vi "ISEG_HVBoardGUI.panel.vi"(0 "object ref":refnum<vi>, 5 "error in (no error)":errorcluster) -> (19 "error out":errorcluster)   [LabVIEW 2014, in "ISEG_HVBoardGUI.lvlib"]
doc: "This is just an example for a ISEG HV Board GUI .\n\nLicense Agreement for this software:\n\nCopyright (C)\nGesellschaft für Schwerionenforschung, GSI\nPlanckstr. 1\n64291 Darmstadt\nGermany\n\nContact: D.Beck@gsi.de \n\nThis program is free software; you can redistribute it and/or modify it under the terms of the GNU General Public License as published by the Free Software Foundation; either version 2 of the license, or (at your option) any later version.\n\nThis program is distributed in the hope that it will be useful, but WITHOUT ANYW ARRANTY; without even the implied warranty of MERCHANTABILITY or FITNESS FOR A PARTICULAR PURPOSE. See the GNU General License for more details (http://www.gnu.org).\n\nGesellschaft für Schwerionenforschung, GSI\nPlanckstr. 1, 64291 Darmstadt, Germany\nFor all questions and ideas contact: M.Richter@gsi.de, H.Brand@gsi.de or D.Beck@gsi.de.\nLast update: 18-DEC-2002"
uses:
  ISEG_HVBoardGUI.lvlib
  CSlibraries-extern/DimLVEvent/DimIndicators/DimIndicators.numericType.ctl
  CSlibraries-extern/DimLVEvent/DimIndicators/DimIndicators.anyType.ctl
  CSCore/CSSystem/CoreDefs/CoreDefs.call_type.ctl
  CSCore/BaseProcess/BaseProcess.descriptor string definition.ctl
  CSCore/CSSystem/CoreDefs/CoreDefs.rawDataType.ctl
  CSCore/CSSystem/CoreLib/CoreLib.double 2 byte array.vi
  CSCore/CSSystem/CoreLib/CoreLib.short 2 byte array.vi
  CSCore/CSSystem/CoreLib/CoreLib.string 2 byte array.vi
  CSlibraries-extern/DimLVEvent/DimIndicators/DimIndicators.lvlib
  CSCore/CSSystem/CSSystemLib/CSSystemLib.lvlib
  CSCore/CSSystem/CoreLib/CoreLib.lvlib
  CSCore/BaseProcess/BaseProcess.lvlib
  CSlibraries/UtilityLib/UtilityLib.lvlib
panel:
  out "Status":bool
  in  "Refresh":T1
  out "Refrech":bool caption="CANBUS_BUSY"
  out "On/Off_Status":bool
  in  "Event_Status":T1
  in  "SetVAll":T1
  in  "On":T1
  in  "Clear":T1
  in  "Kill":T1
  in  "RampRate":T1
  out "Device Class":dbl
  in  "DeviceClass":T1
  in  "AlarmStatus":T1
  in  "Alarm":T1
  in  "Clear":bool
  in  "SetRampRate":dbl
  in  "On":bool
  out "Alarm":bool
  out "AlarmStatus":u16 caption="Alarming" format="%.0b"
  in  "SetV All channels":dbl
  in  "call cluster in":T2={"Object"="", "Selector"="", "CallType"=enum."synchronous", "Async Object"="", "Async Selector"="", "Data Descriptor"="", "Data"=[], "Error #"=0, "Expire"=0}
  in  "KillStatus":T1
  in  "Kill":bool
  out "Status":bool
  in  "BoardTemp":T1
  in  "HardwareVLimit":T1
  in  "Status":T1
  in  "NrOfCh":T1
  in  "DeviceID":T5
  out "loop counter":i32
  in  "DeviceState":T1
  out "Object Name":string
  out "Board":i16
  out "System Name":string
  out "Temp":dbl
  out "NrOfCh":u16
  out "HVMax":dbl format="%#_f"
  out "BdStatus":u16 caption="Status" format="%016b"
  out "DeviceID":string
  out "time stamp":timestamp
  in  "stop":bool
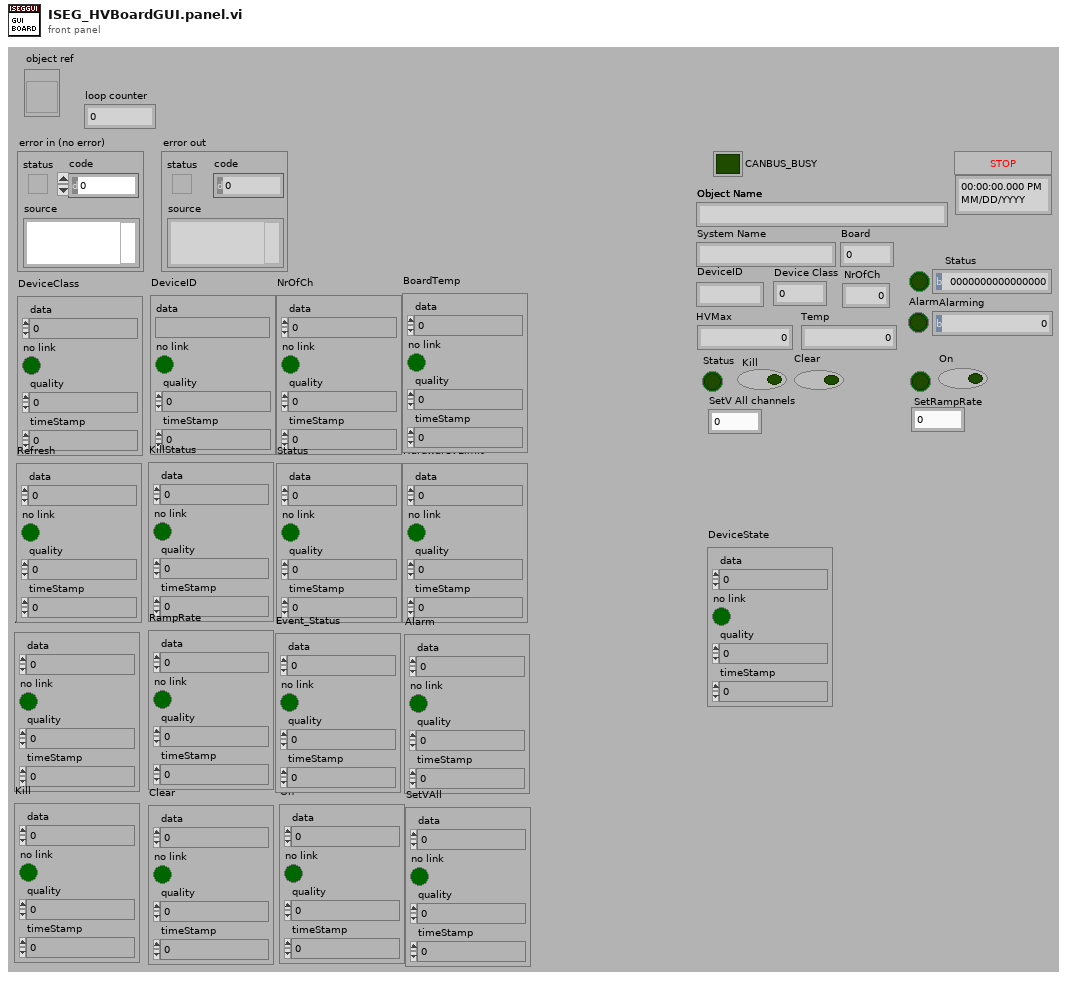
[diagram p1: front panel]
types:
  T1 = typedef "DimIndicators.lvlib/DimIndicators.numericType.ctl" = cluster{"data":dbl, "no link":bool, "quality":i32, "timeStamp":dbl}
  T2 = typedef "CoreDefs.call_type.ctl" = cluster{"Object":string, "Selector":string, "CallType":enum16{"simple", "synchronous", "asynchronous"}, "Async Object":string, "Async Selector":string, "Data Descriptor":T3, "Data":T4, "Error #":i32, "Expire":u32}
  T3 = typedef "BaseProcess.lvlib/BaseProcess.descriptor string definition.ctl" = string
  T4 = typedef "CoreDefs.rawDataType.ctl" = i8[]
  T5 = typedef "DimIndicators.lvlib/DimIndicators.anyType.ctl" = cluster{"data":string, "no link":bool, "quality":i32, "timeStamp":dbl}
  T6 = typedef "ISEG_HVBoardGUI.lvlib/ISEG_HVBoardGUI.i attribute.ctl" = cluster{"System Name":string, "Slot":i16, "Object Name":string, "Prefix":string}
  T7 = typedef "DeviceBase.lvlib/DeviceBase.deviceState.ctl" = i16
  T8 = typedef "UtilityLib.lvlib/UtilityLib.valueStatus.ctl" = enum16{"no info available", "stand by/off", "on", "warning", "alarm/malfunction", "not implemented", "user action required", "important information", "system default", "control default", "indicator default", "button default"}
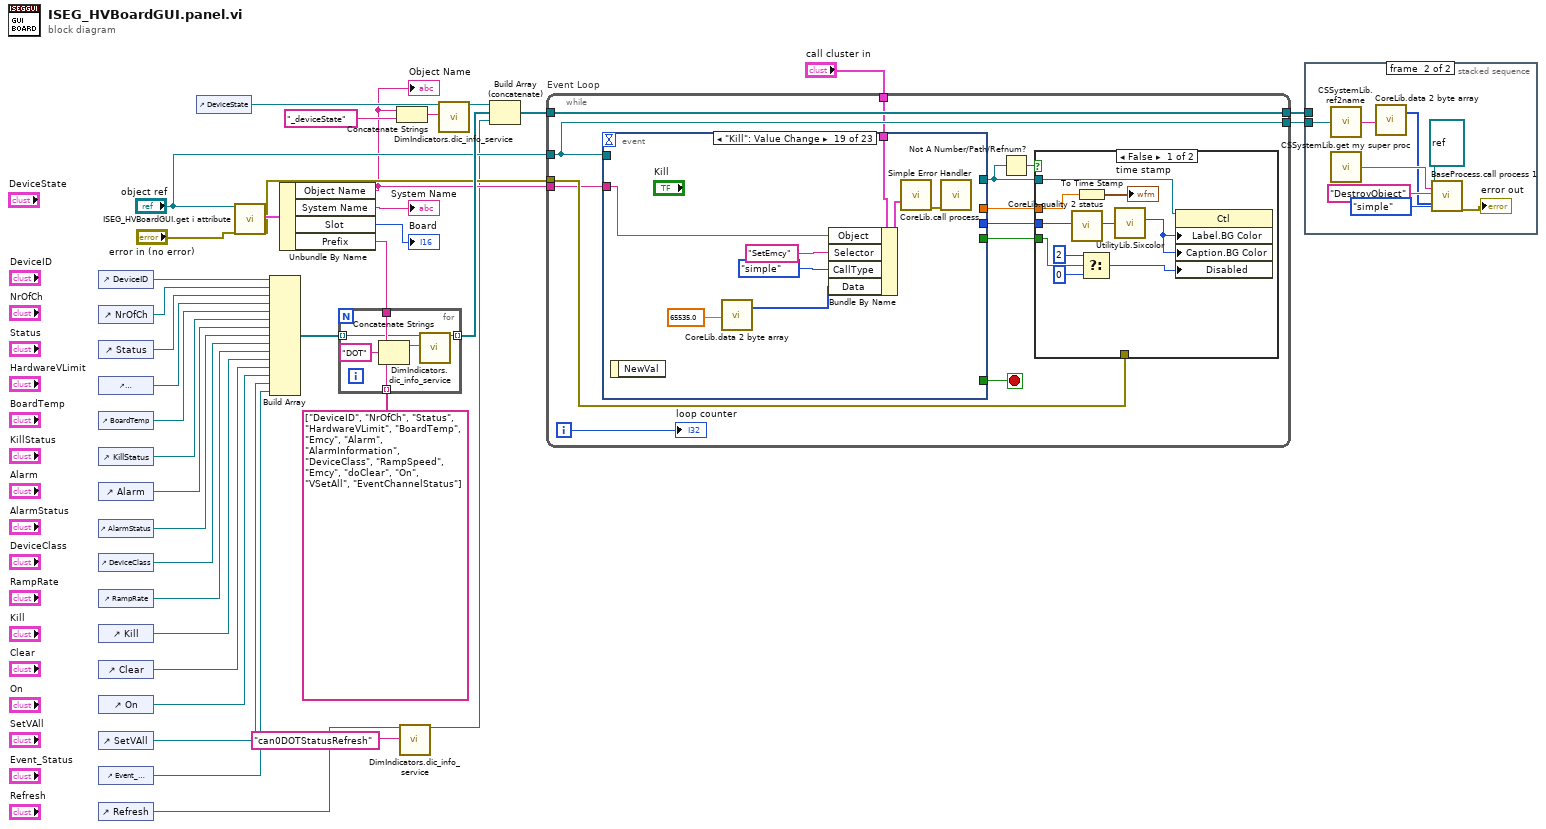
[diagram p0: block diagram]
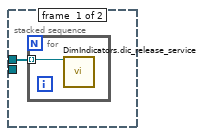
[diagram p2: hidden frame]
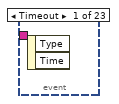
[diagram p4: hidden frame]
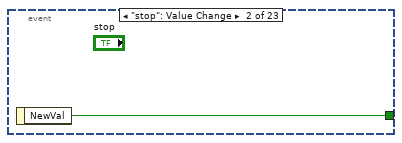
[diagram p5: hidden frame]
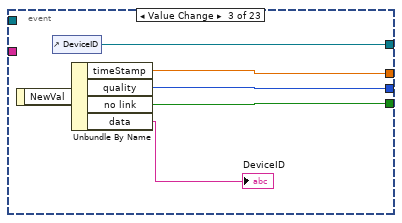
[diagram p6: hidden frame]
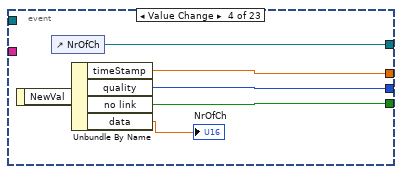
[diagram p7: hidden frame]
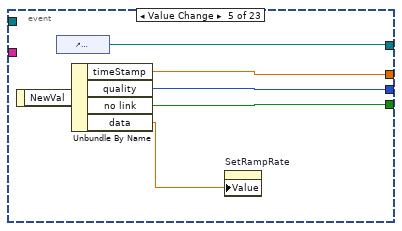
[diagram p8: hidden frame]
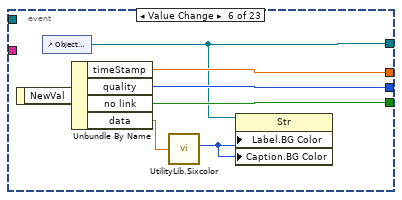
[diagram p9: hidden frame]
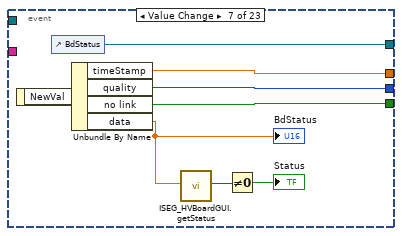
[diagram p10: hidden frame]
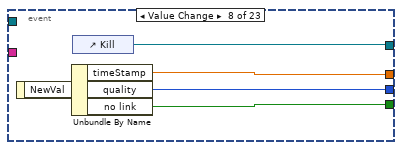
[diagram p11: hidden frame]
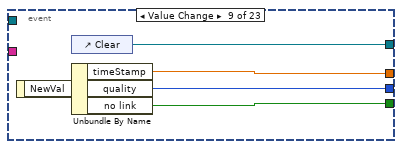
[diagram p12: hidden frame]
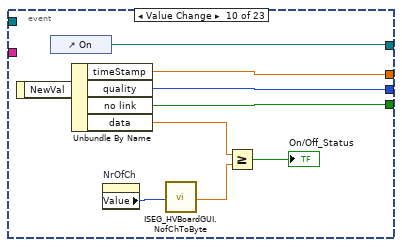
[diagram p13: hidden frame]
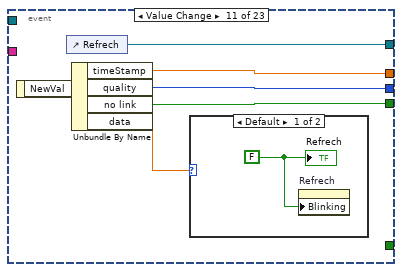
[diagram p14: hidden frame]
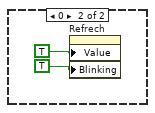
[diagram p15: hidden frame]
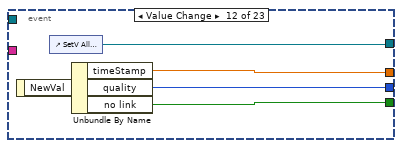
[diagram p16: hidden frame]
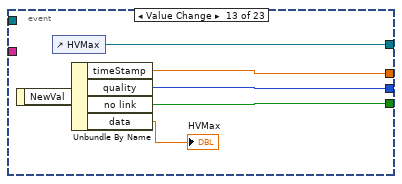
[diagram p17: hidden frame]
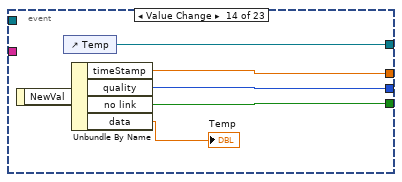
[diagram p18: hidden frame]
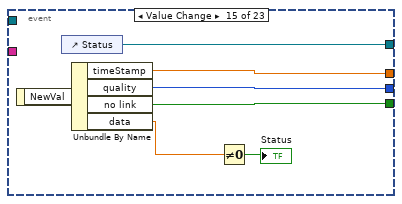
[diagram p19: hidden frame]
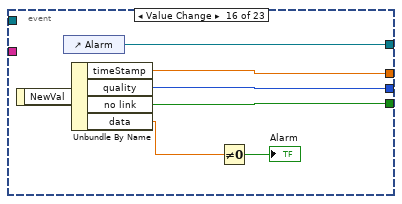
[diagram p20: hidden frame]
diagram:
  n1 = control-ref of="DeviceID"() -> (w29:refnum<vi>)
  n2 = control-ref of="NrOfCh"() -> (w17:refnum<vi>)
  n3 = control-ref of="Status"() -> (w16:refnum<vi>)
  n4 = control-ref of="HardwareVLimit"() -> (w15:refnum<vi>)
  n5 = control-ref of="BoardTemp"() -> (w14:refnum<vi>)
  n6 = control-ref of="KillStatus"() -> (w13:refnum<vi>)
  n7 = control-ref of="Alarm"() -> (w12:refnum<vi>)
  n8 = control-ref of="AlarmStatus"() -> (w11:refnum<vi>)
  n9 = control-ref of="DeviceClass"() -> (w10:refnum<vi>)
  n10 = control-ref of="RampRate"() -> (w9:refnum<vi>)
  n11 = control-ref of="Kill"() -> (w8:refnum<vi>)
  n12 = control-ref of="Clear"() -> (w7:refnum<vi>)
  n13 = control-ref of="On"() -> (w6:refnum<vi>)
  n14 = control-ref of="SetVAll"() -> (w5:refnum<vi>)
  n15 = control-ref of="Event_Status"() -> (w4:refnum<vi>)
  n16 = control-ref of="Refresh"() -> (w2:refnum<vi>)
  n17 = control-ref of="DeviceState"() -> (w31:refnum<vi>)
  n18 = call "ISEG_HVBoardGUI.get i attribute.vi"("i ref in"="object ref", "error in (no error)"="error in (no error)") -> ("i attribute"=w36:T6, "error out"=w22:errorcluster)  [unwired: 15 in, 1 out]
  n19 = Build Array(w29, w17, w16, w15, w14, w13, w12, w11, w10, w9, w8, w7, w6, w5, w4) -> (w28:refnum<vi>[])
  n20 = Unbundle By Name(w36) -> ("Object Name"=w18:string, "System Name"=→"System Name":string, "Slot"=→"Board":i16, "Prefix"=w26:string)
  "Object Name" <- w18
  n21 = for {
    tunnel: w26 -> [w42]
    tunnel: string[] ["DeviceID", "NrOfCh", "Status", "HardwareVLimit", "BoardTemp", "Emcy", "Alarm", "AlarmInformation", "DeviceClass", "RampSpeed", "Emcy", "doClear", "On", "VSetAll", "EventChannelStatus"] -> [w41] mode=indexing
    tunnel: w28 -> [w39] mode=indexing
    tunnel: [w38] -> w25 mode=indexing
    n22 = Concatenate Strings(w42, "DOT" ("string"), w41) -> (w40:string)
    n23 = call "DimIndicators.dic_info_service.vi"("controlRef"=w39, "serviceName"=w40) -> ("controlRef out"=w38:refnum<vi>)  [unwired: 16 in, 1 out]
  }
  n24 = Concatenate Strings(w18, "_deviceState" ("string")) -> (w35:string)
  n25 = call "DimIndicators.dic_info_service.vi"("controlRef"=w2, "serviceName"="can0DOTStatusRefresh") -> ("controlRef out"=w1:refnum<vi>)  [unwired: 16 in, 1 out]
  n26 = call "DimIndicators.dic_info_service.vi"("controlRef"=w31, "serviceName"=w35) -> ("controlRef out"=w30:refnum<vi>)  [unwired: 16 in, 1 out]
  n27 = Build Array (concatenate)(w30, w25, w1) -> (w24:refnum<vi>[])
  n28 = while "Event Loop" {
    tunnel: "object ref" -> [w55]
    tunnel: [w55] -> w20
    tunnel: [w54] -> w21
    tunnel: w24 -> [w54]
    tunnel: w22 -> [w50]
    tunnel: "call cluster in" -> [w45]
    tunnel: w18 -> [w44]
    i -> [w47]
    stop <- w46 stop-if-true
    n29 = event shown="[18] \"Kill\": Value Change" {
      selector: _ -> [_ _ _ _ _ _ _ _ _ _ _ _ _ _ _ _ _ _ _ _ _ _ _]
      dyn-events: _ -> [_ _ _ _ _ _ _ _ _ _ _ _ _ _ _ _ _ _ _ _ _ _ _]
      timeout: _ -> [_ _ _ _ _ _ _ _ _ _ _ _ _ _ _ _ _ _ _ _ _ _ _]
      tunnel: [_ w66 _ _ _ _ _ _ _ _ _ _ _ _ _ _ _ _ _ _ _ _ _] -> w46
      tunnel: w55 -> [_ _ _ _ _ _ _ _ _ _ _ _ _ _ _ _ _ _ _ _ _ _ _]
      tunnel: [_ _ w72 w77 w83 w90 w98 w103 w108 w117 w123 w131 w137 w143 w151 w158 w164 w170 _ _ _ _ _] -> w53
      tunnel: [_ _ w71 w76 w82 w89 w97 w102 w107 w116 w122 w130 w136 w142 w150 w157 w163 w169 _ _ _ _ _] -> w52
      tunnel: [_ _ w67 w73 w79 w87 w95 w100 w105 w114 w120 w128 w133 w139 w147 w153 w160 w165 _ _ _ _ _] -> w49
      tunnel: [_ _ w70 w75 w81 w88 w96 w101 w106 w115 w121 w129 w135 w141 w149 w156 w162 w168 _ _ _ _ _] -> w51
      tunnel: w45 -> [_ _ _ _ _ _ _ _ _ _ _ _ _ _ _ _ _ _ w174 w182 w190 w199 w207]
      tunnel: w44 -> [_ _ _ _ _ _ _ _ _ _ _ _ _ _ _ _ _ _ w173 w181 w189 w198 w206]
      event Timeout {
        n30 = event-data() -> ()  [unwired: 1 in, 2 out]
      }
      event "stop": Value Change {
        n31 = event-data() -> ("NewVal"=w66:bool)  [unwired: 1 in]
      }
      event Value Change {
        n32 = event-data() -> ("NewVal"=w69:T5)  [unwired: 1 in]
        n33 = control-ref of="DeviceID"() -> (w67:refnum<vi>)
        n34 = Unbundle By Name(w69) -> ("timeStamp"=w70:dbl, "quality"=w72:i32, "no link"=w71:bool, "data"=→"DeviceID":string)
      }
      event Value Change {
        n35 = event-data() -> ("NewVal"=w78:T1)  [unwired: 1 in]
        n36 = control-ref of="NrOfCh"() -> (w73:refnum<vi>)
        n37 = Unbundle By Name(w78) -> ("timeStamp"=w75:dbl, "quality"=w77:i32, "no link"=w76:bool, "data"=→"NrOfCh":dbl)
      }
      event Value Change {
        n38 = event-data() -> ("NewVal"=w84:T1)  [unwired: 1 in]
        n39 = control-ref of="SetRampRate"() -> (w79:refnum<vi>)
        n40 = Unbundle By Name(w84) -> ("timeStamp"=w81:dbl, "quality"=w83:i32, "no link"=w82:bool, "data"=w80:dbl)
        n41 = property on="SetRampRate" class="DigNum (strict)"("Value"=w80) -> ()  [unwired: 2 in, 2 out]
      }
      event Value Change {
        n42 = event-data() -> ("NewVal"=w91:T1)  [unwired: 1 in]
        n43 = control-ref of="Object Name"() -> (w87:refnum<vi>)
        n44 = Unbundle By Name(w91) -> ("timeStamp"=w88:dbl, "quality"=w90:i32, "no link"=w89:bool, "data"=w86:dbl)
        n45 = call "UtilityLib.Sixcolor.vi"("State"=w86) -> ("elementBackground"=w85:u32)  [unwired: 2 in, 3 out]
        n46 = property class="Str"(reference=w87, "Label.BG Color"=w85, "Caption.BG Color"=w85) -> ()  [unwired: 1 in, 2 out]
      }
      event Value Change {
        n47 = event-data() -> ("NewVal"=w99:T1)  [unwired: 1 in]
        n48 = control-ref of="BdStatus"() -> (w95:refnum<vi>)
        n49 = Unbundle By Name(w99) -> ("timeStamp"=w96:dbl, "quality"=w98:i32, "no link"=w97:bool, "data"=w94:dbl)
        "BdStatus" <- w94
        n50 = call "ISEG_HVBoardGUI.getStatus.vi"("Numeric"=w94) -> ("s? t:f"=w93:T7)  [unwired: 18 in]
        n51 = Not Equal To 0?(x=w93) -> (x != 0?=→"Status":bool)
      }
      event Value Change {
        n52 = event-data() -> ("NewVal"=w104:T1)  [unwired: 1 in]
        n53 = Unbundle By Name(w104) -> ("timeStamp"=w101:dbl, "quality"=w103:i32, "no link"=w102:bool)
        n54 = control-ref of="Kill"() -> (w100:refnum<vi>)
      }
      event Value Change {
        n55 = event-data() -> ("NewVal"=w109:T1)  [unwired: 1 in]
        n56 = control-ref of="Clear"() -> (w105:refnum<vi>)
        n57 = Unbundle By Name(w109) -> ("timeStamp"=w106:dbl, "quality"=w108:i32, "no link"=w107:bool)
      }
      event Value Change {
        n58 = event-data() -> ("NewVal"=w118:T1)  [unwired: 1 in]
        n59 = control-ref of="On"() -> (w114:refnum<vi>)
        n60 = Unbundle By Name(w118) -> ("timeStamp"=w115:dbl, "quality"=w117:i32, "no link"=w116:bool, "data"=w113:dbl)
        n61 = property on="NrOfCh" class="DigNum (strict)"() -> ("Value"=w111:u16)  [unwired: 2 in, 2 out]
        n62 = call "ISEG_HVBoardGUI.NofChToByte.vi"("NofCh"=w111) -> ("Byte"=w110:dbl)  [unwired: 18 in]
        n63 = Greater Or Equal?(x=w113, y=w110) -> (x >= y?=→"On/Off_Status":bool)
      }
      event Value Change {
        n64 = event-data() -> ("NewVal"=w124:T1)  [unwired: 1 in]
        n65 = control-ref of="Refrech"() -> (w120:refnum<vi>)
        n66 = Unbundle By Name(w124) -> ("timeStamp"=w121:dbl, "quality"=w123:i32, "no link"=w122:bool, "data"=w119:dbl)
        n67 = case shown="Default" w119 {
          frame Default {
            w125 = FALSE
            n68 = property on="Refrech" class="Bool (strict)"("Blinking"=w125) -> ()  [unwired: 2 in, 2 out]
            "Refrech" <- w125
          }
          frame 0 {
            n69 = property on="Refrech" class="Bool (strict)"("Value"=TRUE ("Refrech"), "Blinking"=TRUE) -> ()  [unwired: 2 in, 2 out]
          }
        }
      }
      event Value Change {
        n70 = event-data() -> ("NewVal"=w132:T1)  [unwired: 1 in]
        n71 = control-ref of="SetV All channels"() -> (w128:refnum<vi>)
        n72 = Unbundle By Name(w132) -> ("timeStamp"=w129:dbl, "quality"=w131:i32, "no link"=w130:bool)
      }
      event Value Change {
        n73 = event-data() -> ("NewVal"=w138:T1)  [unwired: 1 in]
        n74 = control-ref of="HVMax"() -> (w133:refnum<vi>)
        n75 = Unbundle By Name(w138) -> ("timeStamp"=w135:dbl, "quality"=w137:i32, "no link"=w136:bool, "data"=→"HVMax":dbl)
      }
      event Value Change {
        n76 = event-data() -> ("NewVal"=w144:T1)  [unwired: 1 in]
        n77 = control-ref of="Temp"() -> (w139:refnum<vi>)
        n78 = Unbundle By Name(w144) -> ("timeStamp"=w141:dbl, "quality"=w143:i32, "no link"=w142:bool, "data"=→"Temp":dbl)
      }
      event Value Change {
        n79 = event-data() -> ("NewVal"=w148:T1)  [unwired: 1 in]
        n80 = control-ref of="Status"() -> (w147:refnum<vi>)
        n81 = Unbundle By Name(w148) -> ("timeStamp"=w149:dbl, "quality"=w151:i32, "no link"=w150:bool, "data"=w146:dbl)
        n82 = Not Equal To 0?(x=w146) -> (x != 0?=→"Status":bool)
      }
      event Value Change {
        n83 = event-data() -> ("NewVal"=w155:T1)  [unwired: 1 in]
        n84 = control-ref of="Alarm"() -> (w153:refnum<vi>)
        n85 = Unbundle By Name(w155) -> ("timeStamp"=w156:dbl, "quality"=w158:i32, "no link"=w157:bool, "data"=w154:dbl)
        n86 = Not Equal To 0?(x=w154) -> (x != 0?=→"Alarm":bool)
      }
      event Value Change {
        n87 = event-data() -> ("NewVal"=w161:T1)  [unwired: 1 in]
        n88 = control-ref of="AlarmStatus"() -> (w160:refnum<vi>)
        n89 = Unbundle By Name(w161) -> ("timeStamp"=w162:dbl, "quality"=w164:i32, "no link"=w163:bool, "data"=→"AlarmStatus":dbl)
      }
      event Value Change {
        n90 = event-data() -> ("NewVal"=w167:T1)  [unwired: 1 in]
        n91 = control-ref of="Device Class"() -> (w165:refnum<vi>)
        n92 = Unbundle By Name(w167) -> ("timeStamp"=w168:dbl, "quality"=w170:i32, "no link"=w169:bool, "data"=→"Device Class":dbl)
      }
      event "Kill": Value Change {
        n93 = event-data() -> ()  [unwired: 1 in, 1 out]
        n94 = call-poly "CoreLib.data 2 byte array.vi"("f64"=65535.0) -> ("byteArray out"=w171:T4)  [unwired: 18 in]
        n95 = Bundle By Name(cluster=w174, "Object"=w173, "Selector"="SetEmcy", "CallType"=enum16{"simple", "synchronous", "asynchronous"}."simple", "Data"=w171) -> (w178:T2)
        n96 = call "CoreLib.call process.vi"("call cluster in"=w178) -> ("error out"=w177:errorcluster)  [unwired: 13 in, 1 out]
        n97 = call <vilib>:"Simple Error Handler.vi"("error in (no error)"=w177) -> ()  [unwired: 4 in, 5 out]
      }
      event "SetV All channels": Value Change {
        n98 = event-data() -> ("NewVal"=w179:dbl)  [unwired: 1 in]
        n99 = call-poly "CoreLib.data 2 byte array.vi"("f64"=w179) -> ("byteArray out"=w180:T4)  [unwired: 18 in]
        n100 = Bundle By Name(cluster=w182, "Object"=w181, "Selector"="VSetAll", "CallType"=enum16{"simple", "synchronous", "asynchronous"}."simple", "Data"=w180) -> (w186:T2)
        n101 = call "CoreLib.call process.vi"("call cluster in"=w186) -> ("error out"=w185:errorcluster)  [unwired: 13 in, 1 out]
        n102 = call <vilib>:"Simple Error Handler.vi"("error in (no error)"=w185) -> ()  [unwired: 4 in, 5 out]
      }
      event "SetRampRate": Value Change {
        n103 = event-data() -> ("NewVal"=w188:dbl)  [unwired: 1 in]
        n104 = call-poly "CoreLib.data 2 byte array.vi"("f64"=w188) -> ("byteArray out"=w187:T4)  [unwired: 18 in]
        n105 = Bundle By Name(cluster=w190, "Object"=w189, "Selector"="SetRampSpeed", "CallType"=enum16{"simple", "synchronous", "asynchronous"}."simple", "Data"=w187) -> (w194:T2)
        n106 = call "CoreLib.call process.vi"("call cluster in"=w194) -> ("error out"=w193:errorcluster)  [unwired: 13 in, 1 out]
        n107 = call <vilib>:"Simple Error Handler.vi"("error in (no error)"=w193) -> ()  [unwired: 4 in, 5 out]
      }
      event "Clear": Value Change {
        n108 = event-data() -> ("NewVal"=w197:bool)  [unwired: 1 in]
        n109 = Boolean To (0,1)(Boolean=w197) -> (0, 1=w196:i16)
        n110 = call-poly "CoreLib.data 2 byte array.vi"("i16"=w196) -> ("byteArray out"=w195:T4)  [unwired: 18 in]
        n111 = Bundle By Name(cluster=w199, "Object"=w198, "Selector"="Clear", "CallType"=enum16{"simple", "synchronous", "asynchronous"}."simple", "Data"=w195) -> (w203:T2)
        n112 = call "CoreLib.call process.vi"("call cluster in"=w203) -> ("error out"=w202:errorcluster)  [unwired: 13 in, 1 out]
        n113 = call <vilib>:"Simple Error Handler.vi"("error in (no error)"=w202) -> ()  [unwired: 4 in, 5 out]
      }
      event "On": Value Change {
        n114 = event-data() -> ()  [unwired: 1 in, 1 out]
        n115 = call-poly "CoreLib.data 2 byte array.vi"("f64"=65535.0) -> ("byteArray out"=w204:T4)  [unwired: 18 in]
        n116 = Bundle By Name(cluster=w207, "Object"=w206, "Selector"="SetOnOff", "CallType"=enum16{"simple", "synchronous", "asynchronous"}."simple", "Data"=w204) -> (w211:T2)
        n117 = call "CoreLib.call process.vi"("call cluster in"=w211) -> ("error out"=w210:errorcluster)  [unwired: 13 in, 1 out]
        n118 = call <vilib>:"Simple Error Handler.vi"("error in (no error)"=w210) -> ()  [unwired: 4 in, 5 out]
      }
    }
    n119 = Not A Number/Path/Refnum?(number/path/refnum=w49) -> (NaN/Path/Refnum?=w48:bool)
    n120 = case shown="False" w48 {
      tunnel: w53 -> [w63 _]
      tunnel: w52 -> [w62 _]
      tunnel: w51 -> [w61 _]
      tunnel: w50 -> [_ _]
      tunnel: w49 -> [w59 _]
      frame False {
        n121 = call "CoreLib.quality 2 status.vi"("quality"=w63) -> ("valueStatus"=w58:T8)  [unwired: 18 in]
        n122 = To Time Stamp(1:w61) -> (0:→"time stamp":timestamp)
        n123 = Select(t=u8 2 ("Disabled"), s=w62, f=u8 0) -> (s? t:f=w56:u8)
        n124 = call "UtilityLib.Sixcolor.vi"("State"=w58) -> ("elementBackground"=w57:u32)  [unwired: 2 in, 3 out]
        n125 = property class="Ctl"(reference=w59, "Label.BG Color"=w57, "Caption.BG Color"=w57, "Disabled"=w56) -> ()  [unwired: 1 in, 2 out]
      }
      frame True {
      }
    }
    "loop counter" <- w47
  }
  n126 = stacked-sequence {
    tunnel: w20 -> [_ w215]
    tunnel: w21 -> [w212 _]
    frame #0 {
      n127 = for {
        tunnel: w212 -> [w213] mode=indexing
        n128 = call "DimIndicators.dic_release_service.vi"("controlRef"=w213) -> ()  [unwired: 18 in, 1 out]
      }
    }
    frame #1 {
      n129 = call "CSSystemLib.ref2name.vi"("obj refnum"=w215) -> ("name"=w219:string)
      n130 = call "CSSystemLib.get my super proc.vi"() -> ("name"=w220:string)  [unwired: 1 in]
      n131 = call-poly "CoreLib.data 2 byte array.vi"("string"=w219) -> ("byteArray out"=w217:T4)  [unwired: 18 in]
      n132 = call "BaseProcess.call process 1.vi"("i ref in"=refnum<vi> refnum, "Object"=w220, "Selector"="DestroyObject", "CallType"=enum16{"simple", "synchronous", "asynchronous"}."simple", "Data"=w217) -> ("error out"=→"error out":errorcluster)  [unwired: 12 in, 2 out]
    }
  }
